vi "readBaseAliasSettings.vi"(8 "error in (no error)":errorcluster, 11 "Boot in":refnum<class "Boot.lvclass">) -> (0 "error out":errorcluster, 2 "SettingAliases":T1, 3 "Boot out":refnum<class "Boot.lvclass">)   [LabVIEW 2016, in "Boot.lvclass"]
uses:
  Boot.lvclass
  DataTypes/Settings/Base/SettingAliases.ctl
  DataTypes/Settings/Base/SettingAlias.ctl
  Boot.lvclass/Boot.ctl
  Settings/Settings/Setting.lvclass
  DataTypes/Settings/M1M3SupportSettings.lvlib
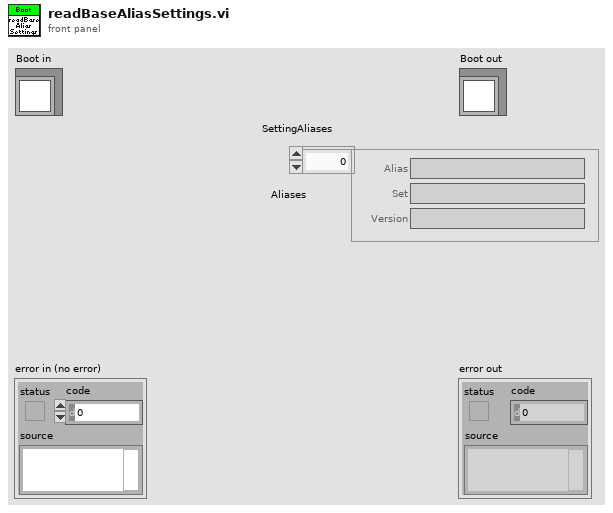
[diagram p1: front panel]
types:
  T1 = typedef "M1M3SupportSettings.lvlib/SettingAliases.ctl" = cluster{"Aliases":T2[]}
  T2 = typedef "M1M3SupportSettings.lvlib/SettingAlias.ctl" = cluster{"Alias":string, "Set":string, "Version":string}
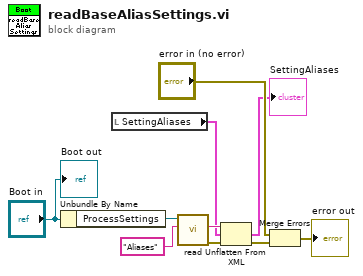
[diagram p0: block diagram]
diagram:
  n1 = Unbundle By Name("Boot in") -> ("ProcessSettings"=w10:refnum<class "Setting.lvclass">)
  n2 = local read "SettingAliases"() -> (w7:T1)
  n3 = call-dynamic "read.vi"("Name"="Aliases", "BaseSetting in"=w10) -> ("error out"=w5:errorcluster, "XML"=w8:string)  [unwired: 6 in, 2 out]
  n4 = Unflatten From XML(xml string=w8, type=w7, error in (no error)=w5) -> (value=→"SettingAliases":T1, error out=w2:errorcluster)
  n5 = Merge Errors("error in (no error)", w2) -> (→"error out":errorcluster)
  "Boot out" <- "Boot in"
